vi "ParseMeasurementsHistory.vi"(11 "Measurements Array":T1[](array[typedef])) -> (2 "Graph Data":dbl[](array[numeric]), 3 "Table Data":string[][](array[string]))   [LabVIEW 2026]
uses:
  MeasurementCluster.ctl
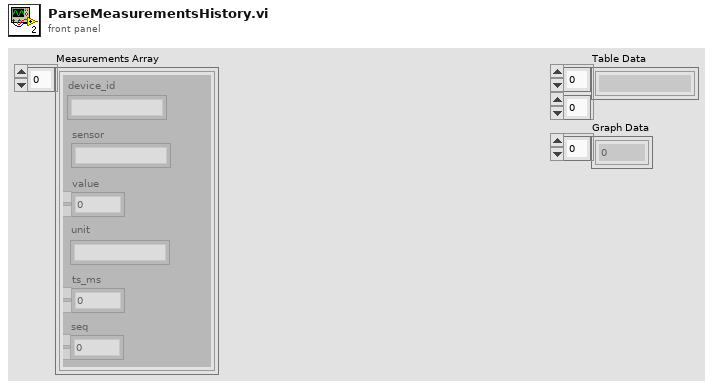
[diagram p1: front panel]
types:
  T1 = typedef "MeasurementCluster.ctl" = cluster{"device_id":string, "sensor":string, "value":dbl, "unit":string, "ts_ms":dbl, "seq":dbl}
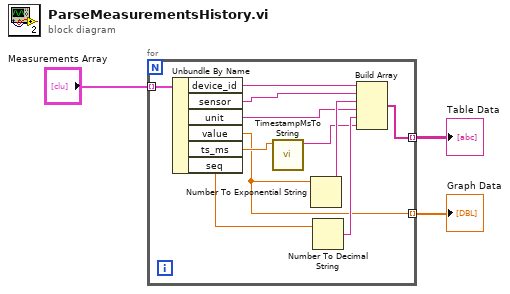
[diagram p0: block diagram]
diagram:
  n1 = for {
    tunnel: [w6] -> w2 mode=indexing
    tunnel: "Measurements Array" -> [w5] mode=indexing
    tunnel: [w4] -> w1 mode=indexing
    n2 = Unbundle By Name(w5) -> ("device_id"=w14:string, "sensor"=w13:string, "unit"=w7:string, "value"=w4:dbl, "ts_ms"=w9:dbl, "seq"=w11:dbl)
    n3 = call "TimestampMsToString.vi"("timestamp_ms"=w9) -> ("timestamp_str"=w8:string)  [unwired: 10 in]
    n4 = Number To Exponential String(number=w4) -> (E-format string=w12:string)  [unwired: 3 in]
    n5 = Number To Decimal String(number=w11) -> (decimal integer string=w10:string)  [unwired: 1 in]
    n6 = Build Array(w14, w13, w12, w7, w10, w8) -> (w6:string[])
  }
  "Table Data" <- w2
  "Graph Data" <- w1
